vi "20TDewar_Manage_Monitor.vi"(4 "System Monitor Variables (in)":T2, 5 "Command (in)":T1={"Dewar Heater (%) Bar"=0.0, "Dewar-Heater (%) Display"=3.4572, "Dewar-Heater (%) SP"=0.0, "Set Dewar-Heater SP"=FALSE, "Change D-Heater Status"=FALSE, "Dewar Pressure"=0.0, "Dewar heater manual"=FALSE, "Dewar Heater (W)"=0.0} {"Dewar Pressure" format="%#4_5f"; "Dewar-Heater (%) Display" format="%4_5g"; "Dewar Heater (%) Bar" scale=0.0..100.0}, 6 "Global Status (in)":T1={"Dewar Heater (%) Bar"=0.0, "Dewar-Heater (%) Display"=3.4572, "Dewar-Heater (%) SP"=0.0, "Set Dewar-Heater SP"=FALSE, "Change D-Heater Status"=FALSE, "Dewar Pressure"=0.0, "Dewar heater manual"=FALSE, "Dewar Heater (W)"=0.0} {"Dewar Pressure" format="%#4_5f"; "Dewar-Heater (%) Display" format="%4_5g"; "Dewar Heater (%) Bar" scale=0.0..100.0}, 7 "queue (in)":refnum<queue>) -> (0 "System Monitor Variables (out)":T2, 1 "Monitor (out)":T1={"Dewar Heater (%) Bar"=0.0, "Dewar-Heater (%) Display"=3.4572, "Dewar-Heater (%) SP"=0.0, "Set Dewar-Heater SP"=FALSE, "Change D-Heater Status"=FALSE, "Dewar Pressure"=0.0, "Dewar heater manual"=FALSE, "Dewar Heater (W)"=0.0} {"Dewar Pressure" format="%#4_5f"; "Dewar-Heater (%) Display" format="%4_5g"; "Dewar Heater (%) Bar" scale=0.0..100.0})   [LabVIEW 2019]
uses:
  Global/Global Variables/System Monitor Cluster.ctl
  Gustav/20T_Dewar_Cluster.ctl
panel:
  # "Dewar Pressure\n(mbar)"
  # "Dewar Heater\nPower (%)"
  # "Dewar Heater\nPower (W)"
  # "20T Dewar"
  # "Dewar Pressure\n(mbar)"
  # "Dewar Heater\nPower (%)"
  # "Dewar Heater\nPower (W)"
  # "20T Dewar"
  # "Dewar Pressure\n(mbar)"
  # "Dewar Heater\nPower (%)"
  # "Dewar Heater\nPower (W)"
  # "20T Dewar"
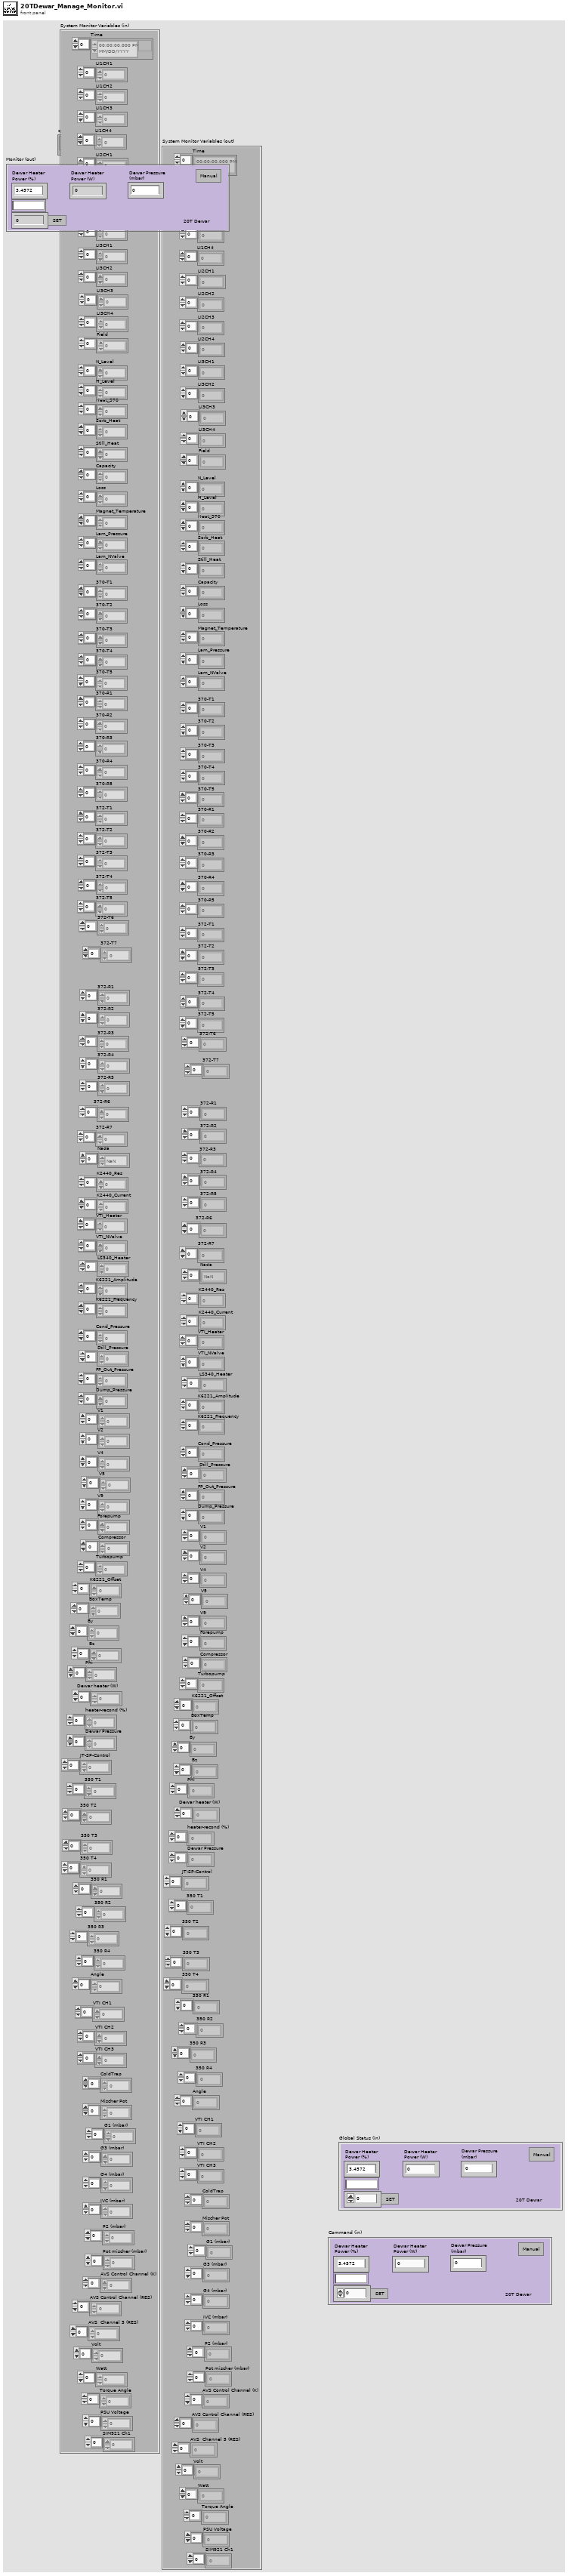
[diagram p1: front panel]
types:
  T1 = typedef "20T_Dewar_Cluster.ctl" = cluster{"Dewar Heater (%) Bar":dbl, "Dewar-Heater (%) Display":dbl, "Dewar-Heater (%) SP":dbl, "Set Dewar-Heater SP":bool, "Change D-Heater Status":bool, "Dewar Pressure":dbl, "Dewar heater manual":bool, "Dewar Heater (W)":dbl}
  T2 = typedef "System Monitor Cluster.ctl" = cluster{"Time":timestamp[], "LI1CH1":dbl[], "LI1CH2":dbl[], "LI2CH1":dbl[], "LI2CH2":dbl[], "LI3CH1":dbl[], "LI3CH2":dbl[], "Field":dbl[], "N_Level":dbl[], "H_Level":dbl[], "Heat_370":dbl[], "Sorb_Heat":dbl[], "Still_Heat":dbl[], "Capacity":dbl[], "Loss":dbl[], "Magnet_Temperature":dbl[], "Lam_Pressure":dbl[], "Lam_NValve":dbl[], "370-T1":dbl[], "370-T2":dbl[], "370-T3":dbl[], "370-T4":dbl[], "370-T5":dbl[], "370-R1":dbl[], "370-R2":dbl[], "370-R3":dbl[], "370-R4":dbl[], "370-R5":dbl[], "372-T1":dbl[], "372-T2":dbl[], "372-T3":dbl[], "372-T4":dbl[], "372-T5":dbl[], "372-T6":dbl[], "372-R1":dbl[], "372-R2":dbl[], "372-R3":dbl[], "372-R4":dbl[], "372-R5":dbl[], "372-R6":dbl[], "Nada":dbl[], "K2440_Res":dbl[], "K2440_Current":dbl[], "VTI_Heater":dbl[], "VTI_NValve":dbl[], "LS340_Heater":dbl[], "K6221_Amplitude":dbl[], "K6221_Frequency":dbl[], "Cond_Pressure":dbl[], "Still_Pressure":dbl[], "FP_Out_Pressure":dbl[], "Dump_Pressure":dbl[], "V1":dbl[], "V2":dbl[], "V4":dbl[], "V5":dbl[], "V9":dbl[], "Forepump":dbl[], "Compressor":dbl[], "K6221_Offset":dbl[], "BoxTemp":dbl[], "By":dbl[], "Bz":dbl[], "Phi":dbl[], "heater-recond (%)":dbl[], "Dewar Pressure ":dbl[], "JT-SP-Control":dbl[], "350 T1":dbl[], "350 T2":dbl[], "350 T3":dbl[], "350 T4":dbl[], "350 R1":dbl[], "350 R2":dbl[], "350 R3":dbl[], "350 R4":dbl[], "Angle":dbl[], "VTI CH1":dbl[], "VTI CH2":dbl[], "VTI CH3":dbl[], "ColdTrap":dbl[], "Mischer Pot":dbl[], "G1 (mbar)":dbl[], "G3 (mbar) ":dbl[], "G4 (mbar)":dbl[], "IVC (mbar)":dbl[], "P2 (mbar) ":dbl[], "Pot mischer (mbar)":dbl[], "AVS Control Channel (K)":dbl[], "AVS Control Channel (RES)":dbl[], "AVS  Channel 5 (RES) ":dbl[], "LI3CH3":dbl[], "LI3CH4":dbl[], "LI1CH3":dbl[], "LI1CH4":dbl[], "LI2CH3":dbl[], "LI2CH4":dbl[], "Volt":dbl[], "Watt":dbl[], "Torque Angle":dbl[], "Dewar heater (W)":dbl[], "PSU Voltage":dbl[], "Turbopump":dbl[], "372-R7":dbl[], "372-T7":dbl[], "SIM921 Ch1":dbl[]}
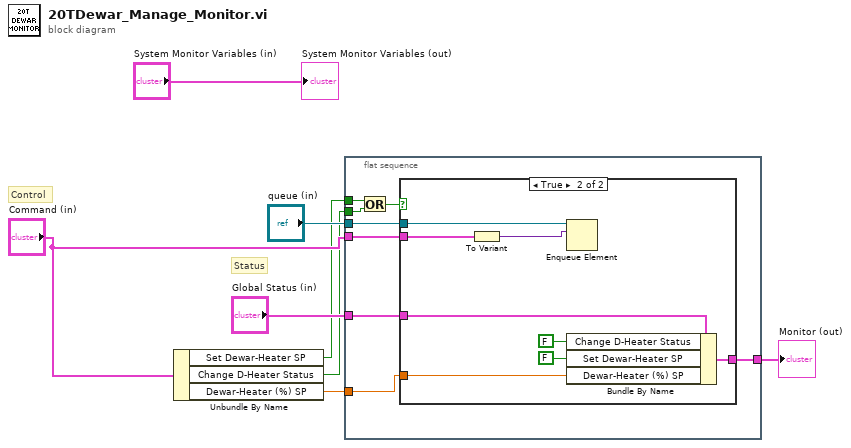
[diagram p0: block diagram]
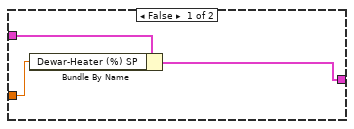
[diagram p2: hidden frame]
diagram:
  # "Status"
  # "Control"
  n1 = Unbundle By Name("Command (in)") -> ("Set Dewar-Heater SP"=w4:bool, "Change D-Heater Status"=w3:bool, "Dewar-Heater (%) SP"=w1:dbl)
  n2 = flat-sequence {
    tunnel: "queue (in)" -> [w16]
    tunnel: "Command (in)" -> [w14]
    tunnel: "Global Status (in)" -> [w15]
    tunnel: w3 -> [w13]
    tunnel: w4 -> [w12]
    tunnel: [w10] -> w2
    tunnel: w1 -> [w9]
    frame #0 {
      n3 = Or(x=w12, y=w13) -> (x .or. y?=w11:bool)
      n4 = case shown="True" w11 {
        tunnel: w16 -> [_ w27]
        tunnel: w14 -> [_ w25]
        tunnel: [w17 w23] -> w10
        tunnel: w15 -> [w19 w24]
        tunnel: w9 -> [w18 w20]
        frame False {
          n5 = Bundle By Name(cluster=w19, "Dewar-Heater (%) SP"=w18) -> (w17:T1)
        }
        frame True {
          n6 = To Variant(anything=w25) -> (Variant=w26:variant)
          n7 = Enqueue Element(queue=w27, element=w26) -> ()  [unwired: 2 in, 3 out]
          n8 = Bundle By Name(cluster=w24, "Change D-Heater Status"=FALSE, "Set Dewar-Heater SP"=FALSE, "Dewar-Heater (%) SP"=w20) -> (w23:T1)
        }
      }
    }
  }
  "System Monitor Variables (out)" <- "System Monitor Variables (in)"
  "Monitor (out)" <- w2
